vi "SunplusDailyWIP.vi"() -> ()   [LabVIEW 2012]
uses:
  <vilib>/addons/database/Auxilliary.llb/DB Tools Cursor Type.ctl
  <vilib>/Utility/NIReport.llb/NI_report.lvclass
  <vilib>/addons/database/Connection.llb/DB Tools Open Connec (Path).vi
  <vilib>/addons/database/Connection.llb/Conn Execute.vi
  <vilib>/addons/database/Recordset.llb/Rec Fetch Recordset Data (R).vi
  <vilib>/addons/database/Recordset.llb/Rec Destroy - Connection.vi
  <vilib>/addons/database/Recordset.llb/Rec Fetch Integer Data (R).vi
  <vilib>/Utility/NIReport.llb/Append Text Table to Report (wrap).vi
  <vilib>/addons/database/_DB Variant To Data/Database Variant To Data.xnode
  <vilib>/addons/database/NI_Database_API.lvlib
  <vilib>/Utility/NIReport.llb/Excel/NI_Excel.lvclass
  <vilib>/Utility/SMTP/NI_SMTPEmail.lvlib
panel:
  in  "template (empty)":path=path "O:/Monitor/Report/SunplusWIP.xls"
  out "array":string[][](array[string])
  out "appended array":string[](array[string])
  out "recordset data":variant[][](array[variant])
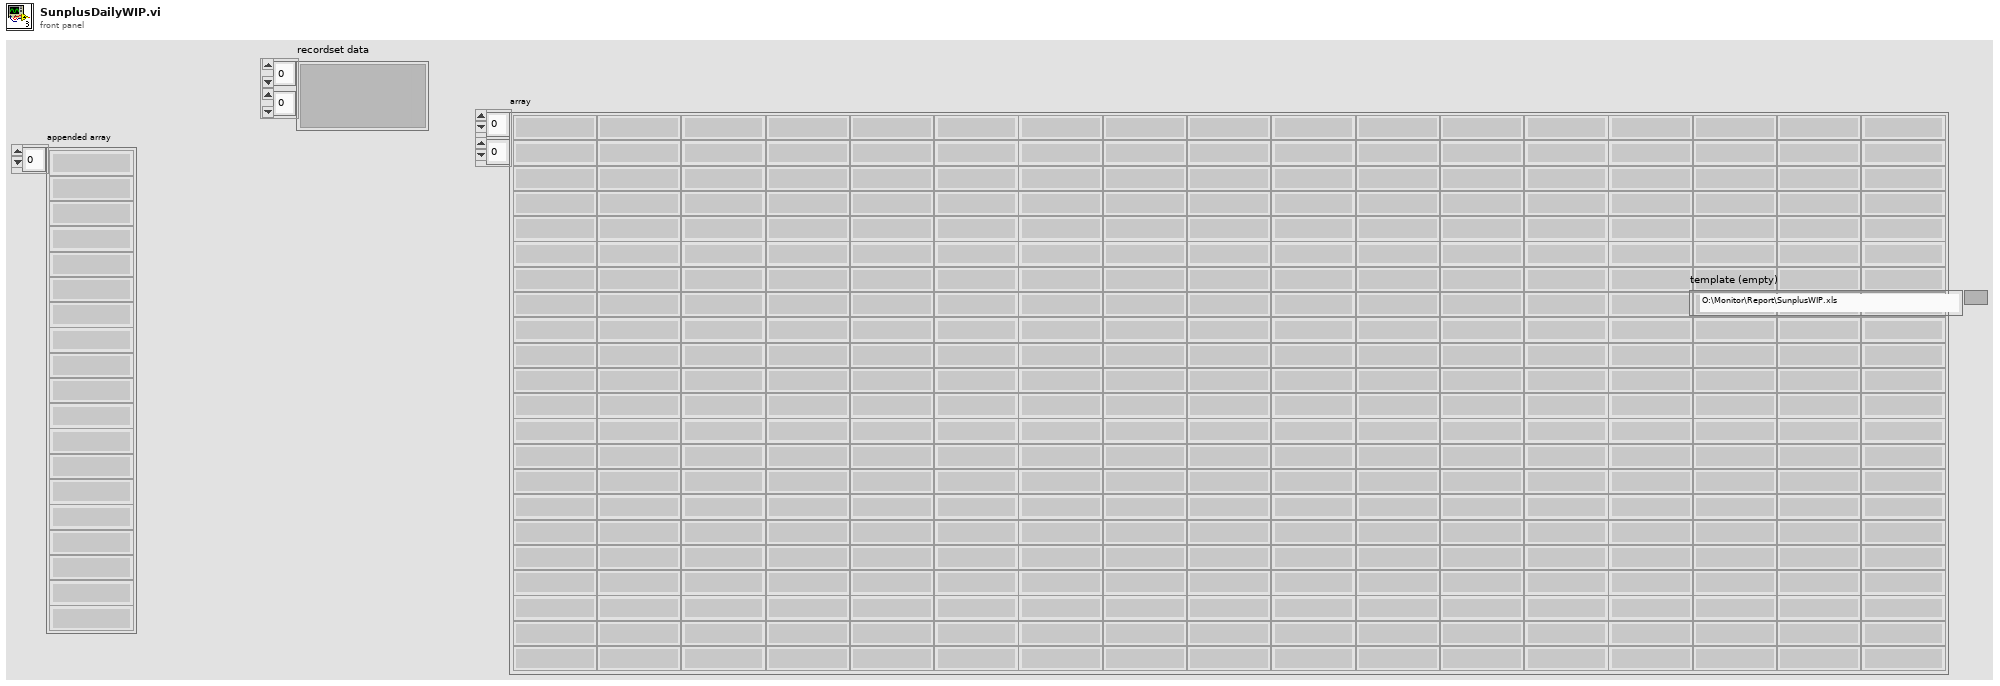
[diagram p1: front panel]
types:
  T1 = typedef "NI_Database_API.lvlib/DB Tools Cursor Type.ctl" = enum16{"forward-only", "keyset", "dynamic", "static"}
  T2 = typedef "NI_Database_API.lvlib/Conn ObjectReference.ctl" = refnum<k1>
  T3 = typedef "NI_Database_API.lvlib/Rec ObjectReference.ctl" = refnum<k1>
  T4 = enum16{"Standard Report", "HTML", "Word", "Excel"}
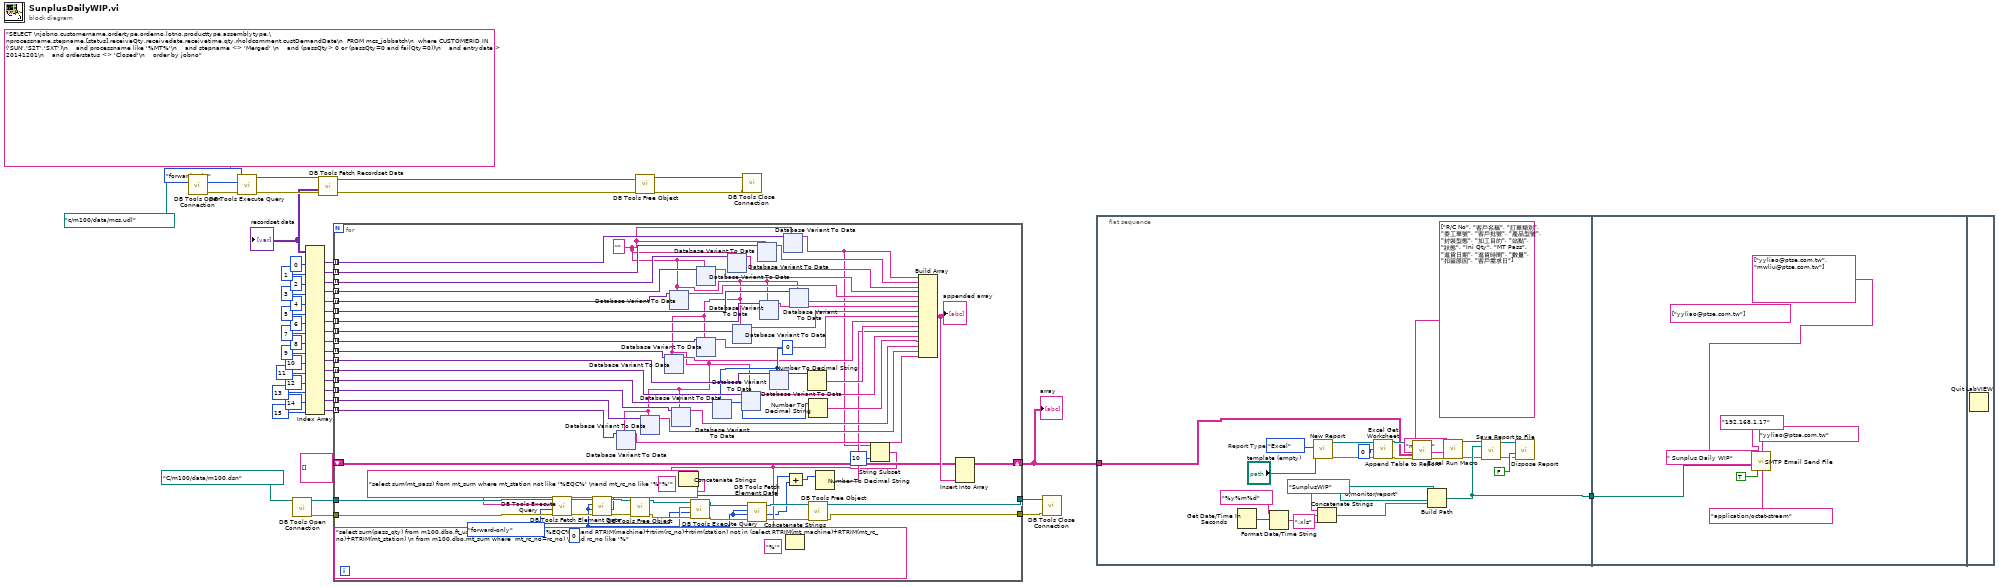
[diagram p0: block diagram]
diagram:
  n1 = call-poly <vilib>:"DB Tools Open Connection.vi"("connection information"=path "c:/m100/data/mcs.udl") -> ("error out"=w51:errorcluster, "connection reference"=w52:T2)  [unwired: 7 in]
  n2 = call-poly <vilib>:"DB Tools Execute Query.vi"("error in (no error)"=w51, "cursor type"=DB_Tools_Cursor_Type."forward-only", "SQL query"="SELECT \njobno,customername,ordertype,orderno,lotno,producttype,assemblytype,\nprocessname,stepname,[status],receiveQty,receivedate,receivetime,qty,rholdcomment,custDemandDate\n  FROM mcs_jobbatch\n  where CUSTOMERID IN ('SUN','S2T','SXT')\n    and processname like '%MT%'\n    and stepname <> 'Merged' \n    and (passQty> 0 or (passQty=0 and failQty=0))\n    and entrydate > 20141201\n    and orderstatus <> 'Closed'\n    order by jobno", "connection reference"=w52) -> ("error out"=w49:errorcluster, "recordset reference"=w50:T3)  [unwired: 4 in]
  n3 = call-poly <vilib>:"DB Tools Open Connection.vi"("connection information"=path "C:/m100/data/m100.dsn") -> ("error out"=w5:errorcluster, "connection reference"=w6:T2)  [unwired: 7 in]
  n4 = call-poly <vilib>:"DB Tools Fetch Recordset Data.vi"("error in (no error)"=w49, "recordset reference"=w50) -> ("error out"=w47:errorcluster, "recordset data"=w41:variant[][], "recordset reference out"=w48:T3)  [unwired: 3 in]
  "recordset data" <- w41
  n5 = Index Array(array=w41, index (col) #1=0 ("disabled index (col)"), index (col) #2=1 ("index (col)"), index (col) #3=2 ("index (col)"), index (col) #4=3 ("index (col)"), index (col) #5=4 ("index (col)"), index (col) #6=5 ("index (col)"), index (col) #7=6 ("index (col)"), index (col) #8=7 ("index (col)"), index (col) #9=8 ("index (col)"), index (col) #10=9 ("index (col)"), index (col) #11=10 ("index (col)"), index (col) #12=11 ("index (col)"), index (col) #13=12 ("index (col)"), index (col) #14=13 ("index (col)"), index (col) #15=14 ("index (col)"), index (col) #16=15 ("index (col)")) -> (element #1=w24:variant[], element #2=w23:variant[], element #3=w22:variant[], element #4=w21:variant[], element #5=w20:variant[], element #6=w19:variant[], element #7=w18:variant[], element #8=w17:variant[], element #9=w16:variant[], element #10=w15:variant[], element #11=w14:variant[], element #12=w13:variant[], element #13=w12:variant[], element #14=w11:variant[], element #15=w10:variant[], element #16=w8:variant[])  [unwired: 16 in]
  n6 = for {
    tunnel: w24 -> [w119] mode=indexing
    tunnel: w23 -> [w118] mode=indexing
    tunnel: w22 -> [w117] mode=indexing
    tunnel: w21 -> [w116] mode=indexing
    tunnel: w20 -> [w115] mode=indexing
    tunnel: w19 -> [w114] mode=indexing
    tunnel: w18 -> [w113] mode=indexing
    tunnel: w17 -> [w112] mode=indexing
    tunnel: w16 -> [w111] mode=indexing
    tunnel: w15 -> [w110] mode=indexing
    tunnel: w14 -> [w109] mode=indexing
    tunnel: w13 -> [w108] mode=indexing
    tunnel: w12 -> [w107] mode=indexing
    tunnel: w11 -> [w106] mode=indexing
    tunnel: w10 -> [w105] mode=indexing
    shift-right: [w87] -> w2
    shift-left: string[][] [] ("array") -> [w86]
    tunnel: w8 -> [w85] mode=indexing
    tunnel: w6 -> [w82]
    tunnel: w5 -> [w81]
    tunnel: [w63] -> w4
    tunnel: [w62] -> w3
    w57 = DB_Tools_Cursor_Type."forward-only" ("cursor type")
    w54 = 0
    w104 = 0
    w84 = ""
    n7 = xnode "Database Variant To Data"("database variant"=w85, "type"=w84) -> ("data"=w83:string)  [unwired: 1 in, 1 out]
    n8 = xnode "Database Variant To Data"("database variant"=w105, "type"=w84) -> ("data"=w89:string)  [unwired: 1 in, 1 out]
    n9 = xnode "Database Variant To Data"("database variant"=w110, "type"=w84) -> ("data"=w95:string)  [unwired: 1 in, 1 out]
    n10 = xnode "Database Variant To Data"("database variant"=w115, "type"=w84) -> ("data"=w100:string)  [unwired: 1 in, 1 out]
    n11 = xnode "Database Variant To Data"("database variant"=w106, "type"=w84) -> ("data"=w90:string)  [unwired: 1 in, 1 out]
    n12 = xnode "Database Variant To Data"("database variant"=w116, "type"=w84) -> ("data"=w101:string)  [unwired: 1 in, 1 out]
    n13 = xnode "Database Variant To Data"("database variant"=w111, "type"=w84) -> ("data"=w96:string)  [unwired: 1 in, 1 out]
    n14 = xnode "Database Variant To Data"("database variant"=w107, "type"=w104) -> ("data"=w92:i32)  [unwired: 1 in, 1 out]
    n15 = xnode "Database Variant To Data"("database variant"=w117, "type"=w84) -> ("data"=w102:string)  [unwired: 1 in, 1 out]
    n16 = xnode "Database Variant To Data"("database variant"=w112, "type"=w84) -> ("data"=w97:string)  [unwired: 1 in, 1 out]
    n17 = xnode "Database Variant To Data"("database variant"=w108, "type"=w84) -> ("data"=w93:string)  [unwired: 1 in, 1 out]
    n18 = xnode "Database Variant To Data"("database variant"=w118, "type"=w84) -> ("data"=w103:string)  [unwired: 1 in, 1 out]
    n19 = xnode "Database Variant To Data"("database variant"=w113, "type"=w84) -> ("data"=w98:string)  [unwired: 1 in, 1 out]
    n20 = xnode "Database Variant To Data"("database variant"=w109, "type"=w104) -> ("data"=w94:i32)  [unwired: 1 in, 1 out]
    n21 = xnode "Database Variant To Data"("database variant"=w119, "type"=w84) -> ("data"=w71:string)  [unwired: 1 in, 1 out]
    n22 = xnode "Database Variant To Data"("database variant"=w114, "type"=w84) -> ("data"=w99:string)  [unwired: 1 in, 1 out]
    n23 = Number To Decimal String(number=w94) -> (decimal integer string=w73:string)  [unwired: 1 in]
    n24 = Number To Decimal String(number=w92) -> (decimal integer string=w91:string)  [unwired: 1 in]
    n25 = String Subset(string=w71, length (rest)=10 ("length (rest)")) -> (substring=w60:string)  [unwired: 1 in]
    n26 = Concatenate Strings("select sum(mt_pass) from mt_sum where mt_station not like '%EQC%' \nand mt_rc_no like '%" ("SQL query"), w60, "%'" ("string")) -> (w74:string)
    n27 = call-poly <vilib>:"DB Tools Execute Query.vi"("error in (no error)"=w81, "cursor type"=w57, "SQL query"=w74, "connection reference"=w82) -> ("error out"=w79:errorcluster, "recordset reference"=w80:T3)  [unwired: 4 in]
    n28 = call-poly <vilib>:"DB Tools Fetch Element Data.vi"("error in (no error)"=w79, "type"=w54, "column index"=w54, "recordset reference"=w80) -> ("error out"=w77:errorcluster, "data"=w55:i32, "recordset reference out"=w78:T3)  [unwired: 3 in]
    n29 = call-poly <vilib>:"DB Tools Free Object.vi"("error in (no error)"=w77, "recordset reference"=w78) -> ("error out"=w68:errorcluster, "connection reference"=w69:T2)  [unwired: 8 in]
    n30 = Concatenate Strings("select sum(pass_qty) from m100.dbo.ft_use where station not like '%EQC%' \nand RTRIM(machine)+rtrim(rc_no)+rtrim(station) not in (select RTRIM(mt_machine)+RTRIM(mt_rc_no)+RTRIM(mt_station) \n from m100.dbo.mt_sum where  mt_rc_no=rc_no) \nand rc_no like '%" ("SQL query"), w60, "%'" ("string")) -> (w58:string)
    n31 = call-poly <vilib>:"DB Tools Execute Query.vi"("error in (no error)"=w68, "cursor type"=w57, "SQL query"=w58, "connection reference"=w69) -> ("error out"=w66:errorcluster, "recordset reference"=w67:T3)  [unwired: 4 in]
    n32 = call-poly <vilib>:"DB Tools Fetch Element Data.vi"("error in (no error)"=w66, "type"=w54, "column index"=w54, "recordset reference"=w67) -> ("error out"=w64:errorcluster, "data"=w53:i32, "recordset reference out"=w65:T3)  [unwired: 3 in]
    n33 = Add(x=w55, y=w53) -> (x+y=w56:i32)
    n34 = call-poly <vilib>:"DB Tools Free Object.vi"("error in (no error)"=w64, "recordset reference"=w65) -> ("error out"=w62:errorcluster, "connection reference"=w63:T2)  [unwired: 8 in]
    n35 = Number To Decimal String(number=w56) -> (decimal integer string=w72:string)  [unwired: 1 in]
    n36 = Build Array(w71, w103, w102, w101, w100, w99, w98, w97, w96, w95, w73, w72, w93, w91, w90, w89, w83) -> (w88:string[])
    "appended array" <- w88
    n37 = Insert Into Array(array=w86, new element=w88) -> (w87:string[][])  [unwired: 2 in]
  }
  "array" <- w2
  n38 = call-poly <vilib>:"DB Tools Free Object.vi"("error in (no error)"=w47, "recordset reference"=w48) -> ("error out"=w45:errorcluster, "connection reference"=w46:T2)  [unwired: 8 in]
  n39 = call <vilib>:"DB Tools Close Connection.vi"("error in (no error)"=w45, "connection reference"=w46) -> ()  [unwired: 5 in, 1 out]
  n40 = call <vilib>:"DB Tools Close Connection.vi"("error in (no error)"=w3, "connection reference"=w4) -> ()  [unwired: 5 in, 1 out]
  n41 = flat-sequence {
    tunnel: w2 -> [w638]
    tunnel: [w637] -> w1
    tunnel: w1 -> [w658]
    frame #0 {
      w656 = T4."Excel"  # Report Type
      n42 = Get Date/Time In Seconds() -> (seconds since 1Jan1904=w643:timestamp)
      n43 = Format Date/Time String(time format string (%c)="%y%m%d", seconds (now)=w643) -> (date/time string=w641:string)  [unwired: 1 in]
      n44 = call <vilib>:"New Report.vi"("report type"=w656, "template (empty)"="template (empty)") -> ("report out"=w655:refnum<class "NI_report.lvclass">, "error out"=w654:errorcluster)  [unwired: 12 in]
      n45 = Concatenate Strings("SunplusWIP" ("string"), w641, ".xls" ("string")) -> (w644:string)
      n46 = call <vilib>:"Excel Get Worksheet.vi"("report in"=w655, "worksheet index (0)"=0, "error in (no error)"=w654) -> ("report out"=w651:refnum<class "NI_report.lvclass">, "error out"=w650:errorcluster)  [unwired: 11 in]
      n47 = call-poly <vilib>:"Append Table to Report.vi"("report in"=w651, "column headers"=string[] ["R/C No", "客戶名稱", "訂單類別", "委工單號", "客戶批號", "產品型號", "封裝型態", "加工目的", "站點", "狀態", "Ini Qty", "MT Pass", "進貨日期", "進貨時間", "數量", "扣留原因", "客戶需求日"], "text data"=w638, "error in (no error)"=w650) -> ("report out"=w633:refnum<class "NI_report.lvclass">, "error out"=w636:errorcluster)  [unwired: 8 in, 2 out]
      n48 = Build Path(base path=path "o:/monitor/report", name or relative path=w644) -> (appended path=w637:path)
      n49 = call <vilib>:"Excel Run Macro.vi"("report in"=w633, "macro name"="macro1", "error in (no error)"=w636) -> ("report out"=w635:refnum<class "NI_report.lvclass">, "error out"=w634:errorcluster)  [unwired: 10 in, 1 out]
      n50 = call-dynamic "Save Report to File.vi"("report in"=w635, "report file path"=w637, "error in (no error)"=w634) -> ("report out"=w648:refnum<class "NI_report.lvclass">, "error out"=w647:errorcluster)  [unwired: 11 in]
      n51 = call-dynamic "Dispose Report.vi"("report in"=w648, "save changes? (F)"=FALSE, "error in (no error)"=w647) -> ()  [unwired: 12 in, 1 out]
    }
    frame #1 {
      (unwired) string[] ["yyliao@ptse.com.tw"] ("recipients")
      n52 = call <vilib>:"SMTP Email Send File.vi"("recipients"=string[] ["yyliao@ptse.com.tw", "mwliu@ptse.com.tw"], "mail server"="192.168.1.17", "return address"="yyliao@ptse.com.tw", "subject ([No Subject])"=" Sunplus Daily WIP", "file path"=w658, "binary? (F)"=TRUE, "MIME content-type (application/octet-stream)"="application/octet-stream") -> ()  [unwired: 7 in, 2 out]
    }
    frame #2 {
      n53 = Quit LabVIEW() -> ()  [unwired: 1 in]
    }
  }
